vi "GEA2 Read ERD.vi"(0 "GEA2 Reference In":refnum<k24>, 1 "Retry Count":i32=5, 2 "Read Timeout (ms)":u32=500, 3 "Expected Data 2":string, 5 "GEA Inputs":T2 {"Destination" format="%.0x"; "Source" format="%.0x"}, 7 "Read ERD List":T3[](array[typedef]) {"ERD Number" format="%.0x"}, 9 "Expected Command 2":string=".*", 11 "Error In":errorcluster, 13 "Verify ERD Response?":bool=TRUE, 14 "Disable Expected Data":bool) -> (4 "GEA2 Reference Out":refnum<k24>, 6 "Raw Data Out":string, 8 "ERD Data Out":T1[](array[typedef]) {"ERD Number" format="%.0x"}, 15 "Error Out":errorcluster)   [LabVIEW 2014, in "GEA2_Toolkit.lvlib"]
doc: "This VI reads an array of ERDs with a single command and returns the data in the data type selected."
uses:
  library/GEA2_Toolkit.lvlib
  C:/Automation/DLLs/PC Tools .NET/GeaCommunication.dll
  Automation/DLLs/PC Tools .NET/GeaCommunication.dll
  type defs/ERD Read Data In.ctl
  type defs/Source_Destination.ctl
  type defs/ERD Read Data Out.ctl
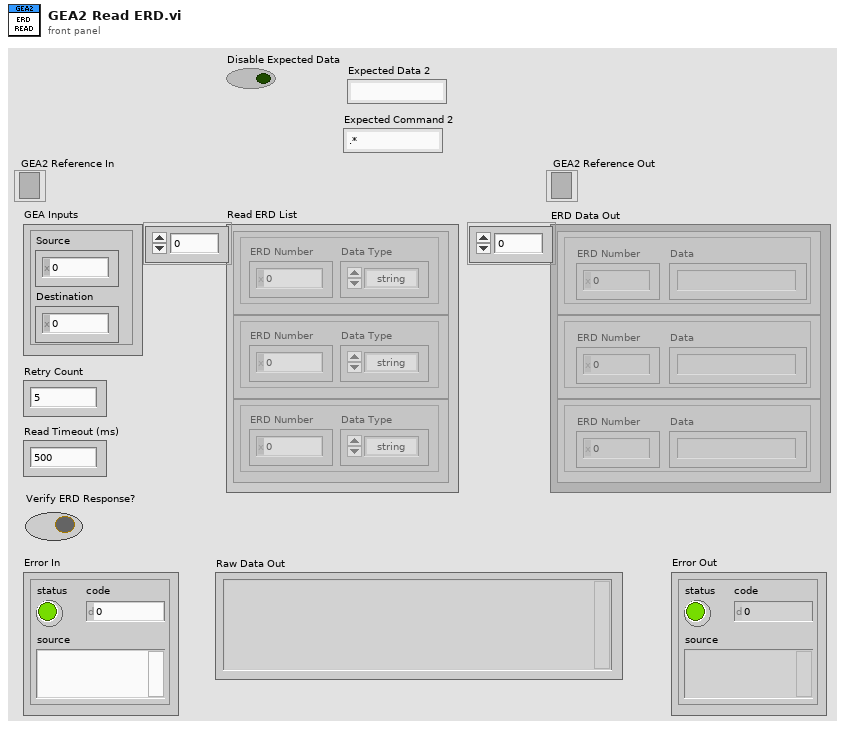
[diagram p1: front panel]
types:
  T1 = typedef "GEA2_Toolkit.lvlib/ERD Read Data Out.ctl" = cluster{"ERD Number":u16, "Data":string}
  T2 = typedef "GEA2_Toolkit.lvlib/Source_Destination.ctl" = cluster{"Source":u8, "Destination":u8}
  T3 = typedef "GEA2_Toolkit.lvlib/ERD Read Data In.ctl" = cluster{"ERD Number":u16, "Data Type":enum16{"string", "boolean", "uint8_t", "uint16_t", "uint32_t", "uint64_t"}}
  T4 = typedef "GEA2_Toolkit.lvlib/Data In.ctl" = cluster{"Source":u8, "Destination":u8, "Command":u8, "Message":string}
  T5 = typedef "GEA2_Toolkit.lvlib/Data Out.ctl" = cluster{"Source":u8, "Destination":u8, "Command":u8, "Length":u8, "CRC":u16, "Message":string}
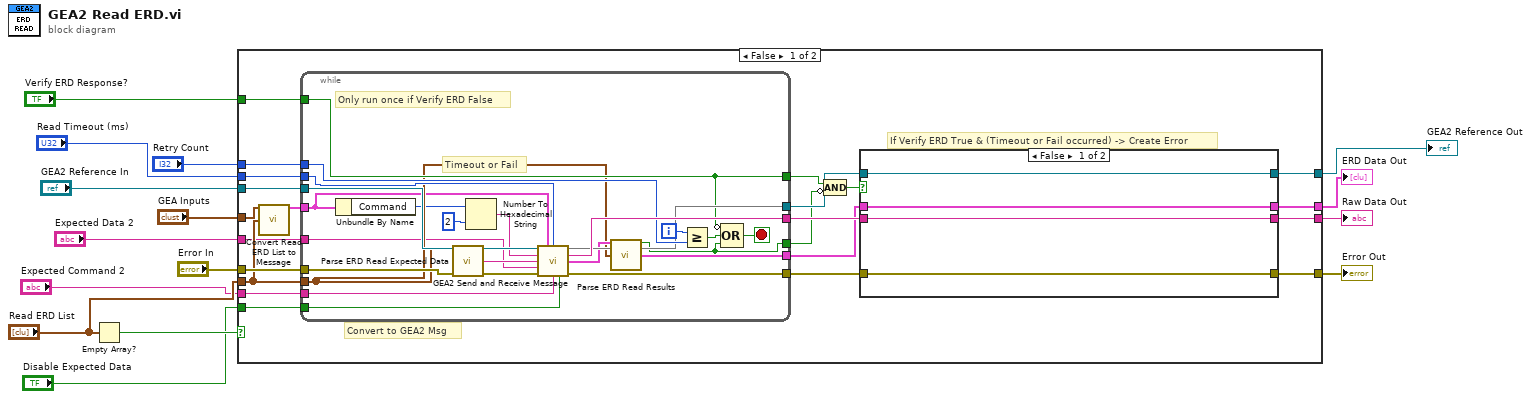
[diagram p0: block diagram]
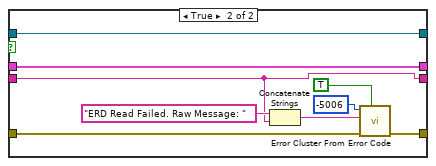
[diagram p2: hidden frame]
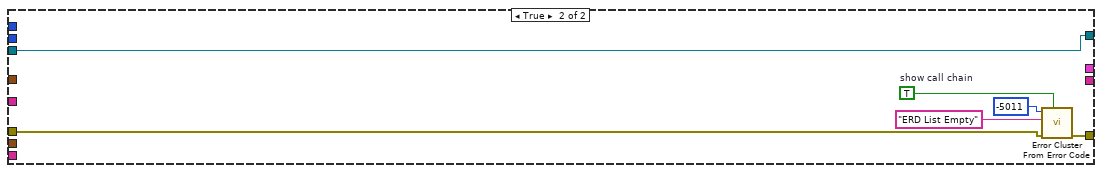
[diagram p3: hidden frame]
diagram:
  n1 = Empty Array?(array="Read ERD List") -> (empty?=w4:bool)
  n2 = case shown="False" w4 {
    tunnel: "Error In" -> [w37 w77]
    tunnel: "GEA2 Reference In" -> [w36 w75]
    tunnel: "GEA Inputs" -> [w35 _]
    tunnel: "Verify ERD Response?" -> [w33 _]
    tunnel: "Read Timeout (ms)" -> [w32 _]
    tunnel: "Retry Count" -> [w31 _]
    tunnel: [w29 w76] -> w9
    tunnel: [w28 _] -> w10
    tunnel: [w25 w75] -> w6
    tunnel: [w24 _] -> w5
    tunnel: "Read ERD List" -> [w21 _]
    tunnel: "Expected Command 2" -> [w18 _]
    tunnel: "Disable Expected Data" -> [w17 _]
    tunnel: "Expected Data 2" -> [w16 _]
    frame False {
      # "If Verify ERD True & (Timeout or Fail occurred) -> Create Error"
      # "Convert to GEA2 Msg"
      n3 = call "Convert Read ERD List to Message.vi"("GEA Inputs"=w35, "Read ERD List"=w21) -> ("GEA Message"=w34:T4)  [unwired: 12 in, 1 out]
      n4 = while {
        tunnel: w37 -> [w66]
        tunnel: w36 -> [w64]
        tunnel: w34 -> [w59]
        tunnel: [w74] -> w27
        tunnel: [w73] -> w30
        tunnel: w33 -> [w67]
        tunnel: w21 -> [w60]
        tunnel: [w62] -> w23
        tunnel: w32 -> [w72]
        tunnel: w31 -> [w70]
        tunnel: [w68] -> w26
        tunnel: [w67] -> w20
        tunnel: [w54] -> w19
        tunnel: w18 -> [w53]
        tunnel: w17 -> [w52]
        tunnel: w16 -> [w51]
        i -> [w71]
        stop <- w69 stop-if-true
        # "Only run once if Verify ERD False"
        # "Timeout or Fail"
        n5 = Unbundle By Name(w59) -> ("Command"=w58:u8)
        n6 = call "Parse ERD Read Expected Data.vi"("Read ERD List"=w60, "Error In"=w66) -> ("Expected Data"=w63:string, "Error Out"=w65:errorcluster)  [unwired: 12 in]
        n7 = Number To Hexadecimal String(1:i16 2 ("width (-)"), 2:w58) -> (0:w56:string)
        n8 = call "GEA2 Send and Receive Message.vi"(0:w64, "Input Data"=w59, "Read Timeout (ms)"=w72, "Expected Command"=w56, "Expected Data"=w63, "Expected Data 2"=w51, "Error In"=w65, "Expected Command 2"=w53, "Disable Expected Data"=w52) -> (4:w68, "Raw Data Out"=w74:string, "Converted Data Out"=w61:T5, "Error Out"=w73:errorcluster)  [unwired: 3 in]
        n9 = call "Parse ERD Read Results.vi"("Converted Data"=w61, "Read ERD List"=w60) -> ("Pass/Fail?"=w54:bool, "ERD Data Out"=w62:T1[])  [unwired: 12 in]
        n10 = Greater Or Equal?(x=w71, y=w70) -> (x >= y?=w55:bool)
        n11 = Compound Arithmetic op=OR(invert w67, w55, w54) -> (w69:bool)
      }
      n12 = Compound Arithmetic op=AND(w20, invert w19) -> (w22:bool)
      n13 = case shown="False" w22 {
        tunnel: w30 -> [w41 w50]
        tunnel: [w41 w49] -> w29
        tunnel: [w40 w43] -> w28
        tunnel: w27 -> [w40 w43]
        tunnel: w26 -> [w39 w46]
        tunnel: [w39 w46] -> w25
        tunnel: [w38 w42] -> w24
        tunnel: w23 -> [w38 w42]
        frame False {
        }
        frame True {
          n14 = Concatenate Strings("ERD Read Failed. Raw Message: " ("error message (\"\")"), w43) -> (w44:string)
          n15 = call <vilib>:"Error Cluster From Error Code.vi"("show call chain? (False)"=TRUE, "error in (no error)"=w50, "error message (\"\")"=w44, "error code (0)"=-5006) -> ("error out"=w49:errorcluster)  [unwired: 5 in]
        }
      }
    }
    frame True {
      w78 = TRUE  # show call chain
      n16 = call <vilib>:"Error Cluster From Error Code.vi"("show call chain? (False)"=w78, "error in (no error)"=w77, "error message (\"\")"="ERD List Empty" ("error message (\"\")"), "error code (0)"=-5011) -> ("error out"=w76:errorcluster)  [unwired: 5 in]
    }
  }
  "Raw Data Out" <- w10
  "Error Out" <- w9
  "GEA2 Reference Out" <- w6
  "ERD Data Out" <- w5
